vi "GetJoystickDrivingData.vi"(8 "error in (no error)":errorcluster, 11 "Refnum in":refnum<k1>) -> (0 "error out":errorcluster, 1 "data string":string, 2 "appended array":T1, 3 "Refnum out":refnum<k1>, 4 "Boolean":bool, 5 "Array":u8[](array[numeric]))   [LabVIEW 2017]
uses:
  TypeDefinitions/Sobot Driving Data.ctl
  <vilib>/Utility/inputDevices.llb/joystickAcquire.vi
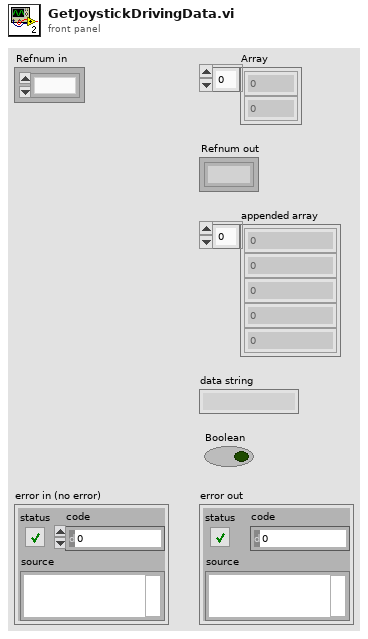
[diagram p1: front panel]
types:
  T1 = typedef "Sobot Driving Data.ctl" = u8[]
  T2 = cluster{"X axis":i32, "Y axis":i32, "Z axis":i32, "X axis rotation":i32, "Y axis rotation":i32, "Z axis rotation":i32, "U axis":i32, "V axis":i32}
  T3 = cluster{"button 1":bool, "button 2":bool, "button 3":bool, "button 4":bool, "button 5":bool, "button 6":bool, "button 7":bool, "button 8":bool, "button 9":bool, "button 10":bool, "button 11":bool, "button 12":bool, "button 13":bool, "button 14":bool, "button 15":bool, "button 16":bool, "button 17":bool, "button 18":bool, "button 19":bool, "button 20":bool, "button 21":bool, "button 22":bool, "button 23":bool, "button 24":bool, "button 25":bool, "button 26":bool, "button 27":bool, "button 28":bool, "button 29":bool, "button 30":bool, "button 31":bool, "button 32":bool}
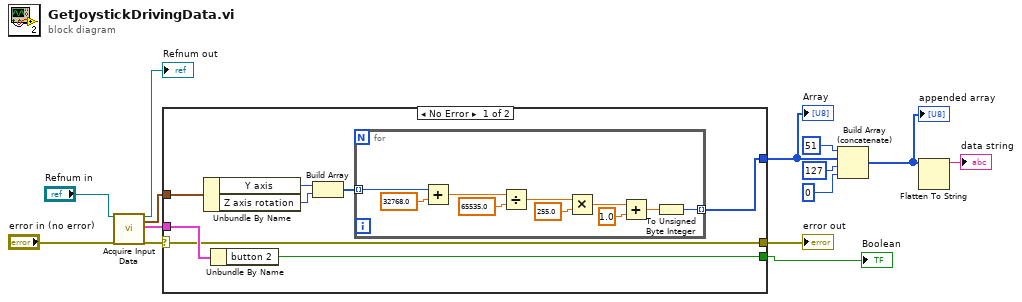
[diagram p0: block diagram]
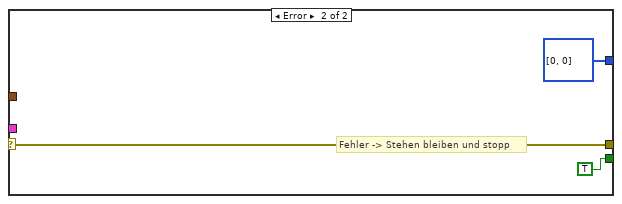
[diagram p2: hidden frame]
diagram:
  n1 = call-poly <vilib>:"Acquire Input Data.vi"("device ID"="Refnum in", "error in (no error)"="error in (no error)") -> ("device ID"=→"Refnum out":refnum<k1>, "axis info"=w4:T2, "button info"=w5:T3, "error out"=w11:errorcluster)  [unwired: 13 in, 1 out]
  n2 = case shown="No Error" w11 {
    selector: w11 -> [w15 w33]
    tunnel: w4 -> [w22 _]
    tunnel: w5 -> [w18 _]
    tunnel: [w17 TRUE ("button 2")] -> w1
    tunnel: [w16 u8[] [0, 0]] -> w6
    tunnel: [w15 w33] -> w14
    frame No Error {
      n3 = Unbundle By Name(w22) -> ("Y axis"=w21:i32, "Z axis rotation"=w20:i32)
      n4 = Unbundle By Name(w18) -> ("button 2"=w17:bool)
      n5 = Build Array(w21, w20) -> (w19:i32[])
      n6 = for {
        tunnel: w19 -> [w31] mode=indexing
        tunnel: [w23] -> w16 mode=indexing
        n7 = Add(x=w31, y=32768.0) -> (x+y=w30:dbl)
        n8 = Divide(x=w30, y=65535.0) -> (x/y=w28:dbl)
        n9 = Multiply(x=w28, y=255.0) -> (x*y=w26:dbl)
        n10 = Add(x=w26, y=1.0) -> (x+y=w24:dbl)
        n11 = To Unsigned Byte Integer(number=w24) -> (unsigned 8bit integer=w23:u8)
      }
    }
    frame Error {
      # "Fehler -> Stehen bleiben und stopp"
    }
  }
  "Array" <- w6
  "error out" <- w14
  "Boolean" <- w1
  n12 = Build Array (concatenate)(u8 51, w6, u8 127, u8 0) -> (w10:u8[])
  "appended array" <- w10
  n13 = Flatten To String(anything=w10) -> (data string=→"data string":string)  [unwired: 3 in, 2 out]
